vi "Find One Cycle R2.vi"(11 "data in":i32[][](array[numeric])) -> (1 "n crossings":i32, 3 "data out":i32[][](array[numeric]))   [LabVIEW 2018]
uses:
  <vilib>/ptbypt/NI_PtbyPt.lvlib
panel:
  out "Array":i32[](array[numeric])
  in  "Trigger":enum16{"either", "minus-plus", "plus-minus"}(ring)
  out "crossing indices":i32[](array[numeric])
  out "Plotting Data":i32[](graph) caption="Waveform Chart - dark"
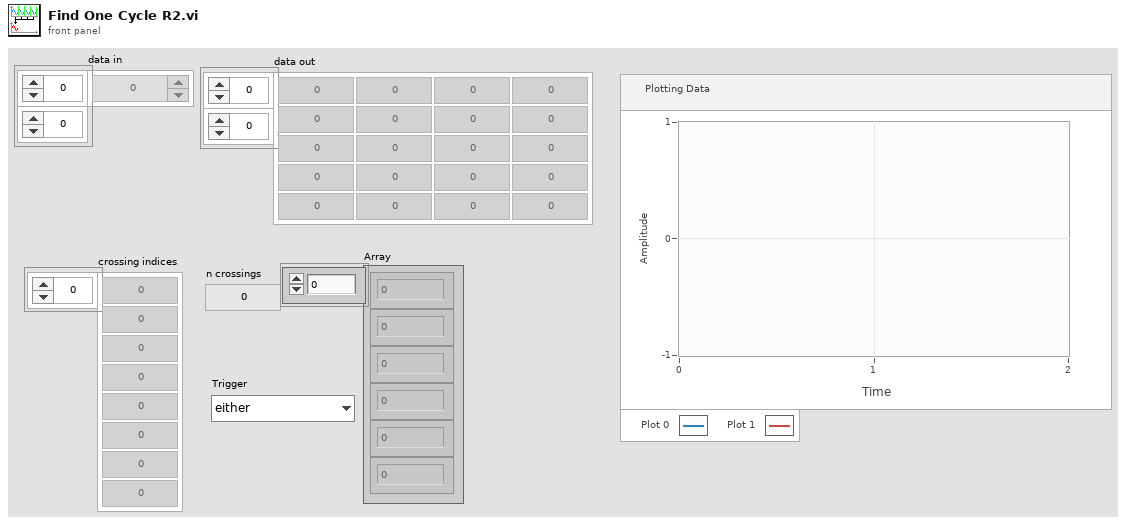
[diagram p1: front panel]
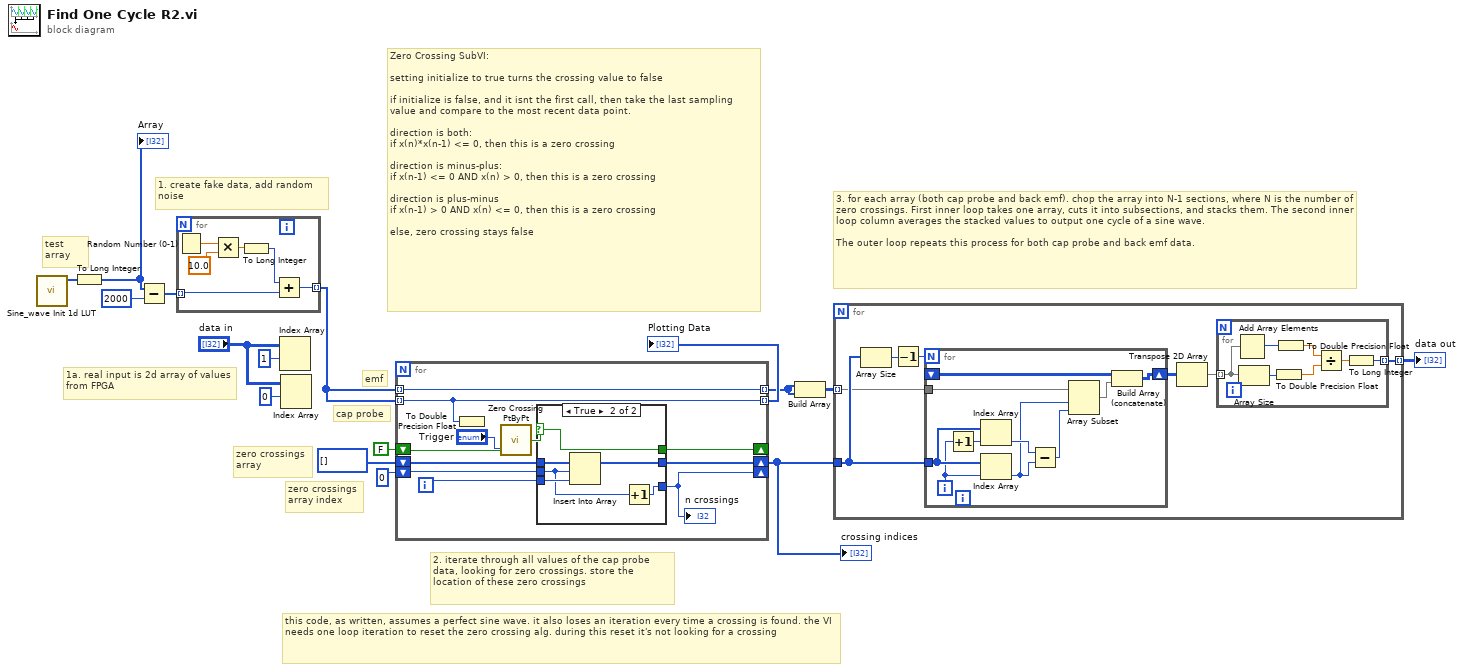
[diagram p0: block diagram]
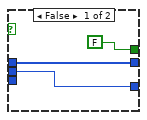
[diagram p2: hidden frame]
diagram:
  # "3. for each array (both cap probe and back emf). chop the array into N-1 sections, where N is the number of zero crossings. First inner loop takes one array, cuts it into subsections, and stacks them. The second inner loop column averages the stacked values to output one cycle of a sine wave.\n\nThe outer loop repeats this process for both cap probe and back emf data."
  # "2. iterate through all values of the cap probe data, looking for zero crossings. store the location of these zero crossings"
  # "1a. real input is 2d array of values from FPGA"
  # "1. create fake data, add random noise"
  # "Zero Crossing SubVI:\n\nsetting initialize to true turns the crossing value to false\n\nif initialize is false, and it isnt the first call, then take the last sampling value and compare to the most recent data point.\n\ndirection is both:\nif x(n)*x(n-1) <= 0, then this is a zero crossing\n\ndirection is minus-plus:\nif x(n-1) <= 0 AND x(n) > 0, then this is a zero crossing\n\ndirection is plus-minus\nif x(n-1) > 0 AND x(n) <= 0, then this is a zero crossing\n\nelse, zero crossing stays false"
  # "test\narray"
  # "cap probe"
  # "emf"
  # "zero crossings\narray index"
  # "zero crossings\narray"
  # "this code, as written, assumes a perfect sine wave. it also loses an iteration every time a crossing is found. the VI needs one loop iteration to reset the zero crossing alg. during this reset it's not looking for a crossing"
  n1 = call "Sine_wave Init 1d LUT.vi"() -> ("Init Data Out"=w2:u16[])  [unwired: 11 in]
  n2 = To Long Integer(number=w2) -> (32bit integer=w1:i32[])
  "Array" <- w1
  n3 = Subtract(x=w1, y=2000 ("index (row)")) -> (x-y=w7:i32[])
  n4 = for {
    tunnel: w7 -> [w18] mode=indexing
    tunnel: [w17] -> w6 mode=indexing
    n5 = Random Number (0-1)() -> (number: 0 to 1=w22:dbl)
    n6 = Multiply(x=w22, y=10.0 ("index (row)")) -> (x*y=w20:dbl)
    n7 = To Long Integer(number=w20) -> (32bit integer=w19:i32)
    n8 = Add(x=w19, y=w18) -> (x+y=w17:i32)
  }
  n9 = Index Array(array="data in", index (row)=1) -> ()  [unwired: 1 in, 1 out]
  n10 = Index Array(array="data in", index (row)=0) -> ()  [unwired: 1 in, 1 out]
  n11 = for {
    shift-right: [w33] -> w8
    shift-left: i32[] [] ("subarray") -> [w31]
    shift-right: [w28] -> _
    shift-left: 0 ("n cycles") -> [w32]
    shift-right: [w29] -> _
    shift-left: FALSE -> [w24]
    tunnel: w6 -> [w30] mode=indexing
    tunnel: [w30] -> w5 mode=indexing
    tunnel: w6 -> [w26] mode=indexing
    tunnel: [w26] -> w9 mode=indexing
    i -> [w27]
    n12 = To Double Precision Float(number=w26) -> ()  [unwired: 1 out]
    n13 = call <vilib>:"Zero Crossing PtByPt.vi"("initialize"=w24, "direction"="Trigger") -> ("crossing"=w23:bool)  [unwired: 1 in]
    n14 = case shown="True" w23 {
      selector: w23 -> [_ w39]
      tunnel: [w36 w42] -> w28
      tunnel: [w35 w40] -> w33
      tunnel: w32 -> [w36 w37]
      tunnel: w31 -> [w35 w41]
      tunnel: [FALSE w39] -> w29
      tunnel: w27 -> [_ w38]
      frame False {
      }
      frame True {
        n15 = Insert Into Array(array=w41, index=w37, new element=w38) -> (w40:i32[])
        n16 = Increment(x=w37) -> (x+1=w42:i32)
      }
    }
    "n crossings" <- w28
  }
  "Plotting Data" <- w9
  "crossing indices" <- w8
  n17 = Build Array(w5, w5) -> (w4:i32[][])
  n18 = for {
    tunnel: w8 -> [w47]
    tunnel: w4 -> [w44] mode=indexing
    tunnel: [w43] -> w3 mode=indexing
    n19 = Array Size(array=w47) -> (size(s)=w49:i32)
    n20 = Decrement(x=w49) -> (x-1=w48:i32)
    n21 = for {
      N: w48 -> [_]
      tunnel: w44 -> [w66]
      shift-right: [w57] -> w45
      shift-left: _ -> [w58]
      tunnel: w47 -> [w65]
      i -> [w64]
      n22 = Increment(x=w64) -> (x+1=w63:i32)
      n23 = Index Array(array=w65, index=w63) -> (element=w61:i32)
      n24 = Index Array(array=w65, index=w64) -> (element=w60:i32)
      n25 = Subtract(x=w61, y=w60) -> (x-y=w62:i32)
      n26 = Array Subset(array=w66, index=w60, length=w62) -> (w59:i32[])
      n27 = Build Array (concatenate)(w58, w59) -> (w57:i32[][])
    }
    n28 = Transpose 2D Array(2D array=w45) -> (transposed array=w46:i32[][])
    n29 = for {
      tunnel: w46 -> [w56] mode=indexing
      tunnel: [w50] -> w43 mode=indexing
      n30 = Add Array Elements(numeric array=w56) -> (sum=w55:i32)
      n31 = Array Size(array=w56) -> (size(s)=w54:i32)
      n32 = To Double Precision Float(number=w54) -> (double precision float=w53:dbl)
      n33 = To Double Precision Float(number=w55) -> (double precision float=w52:dbl)
      n34 = Divide(x=w52, y=w53) -> (x/y=w51:dbl)
      n35 = To Long Integer(number=w51) -> (32bit integer=w50:i32)
    }
  }
  "data out" <- w3
